vi "Get LogFile Path from SysDef.vi"(8 "error in (no error)":errorcluster, 11 "System Definition File":path) -> (0 "error out":errorcluster, 3 "Log File Path":path)   [LabVIEW 2026, in "Telemetry Test Utilities.lvlib"]
uses:
  Telemetry Test Utilities.lvlib
  Source/Shared/Constants.vi
  <vilib>/NI VeriStand/Custom Device Tools/Custom Device Utility Library/NI VeriStand - Search for Item by GUID.vi
  <vilib>/NI VeriStand/Custom Device API/Get Item Property (String Array).vi
  Source/Shared/Telemetry Shared.lvlib
  <vilib>/NI VeriStand/Custom Device Tools/Custom Device Utility Library/Custom Device Utility Library.lvlib
  <vilib>/NI VeriStand/Custom Device API/Custom Device API.lvlib
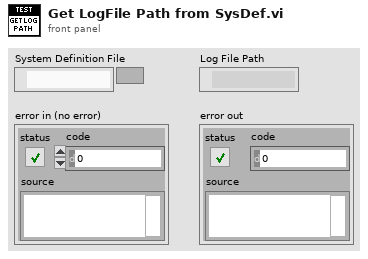
[diagram p1: front panel]
types:
  T1 = typedef "Custom Device API.lvlib/Custom Device Item Ref.ctl" = u64
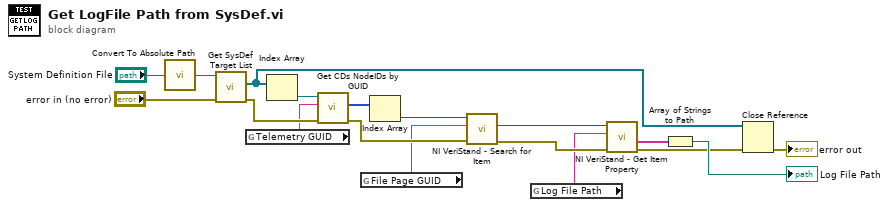
[diagram p0: block diagram]
diagram:
  n1 = call "Convert To Absolute Path.vi"("System Definition File Path"="System Definition File") -> ("Absolute path"=w4:path)
  n2 = call "Get SysDef Target List.vi"("error in (no error)"="error in (no error)", "System Definition Path"=w4) -> ("error out"=w14:errorcluster, "Target List"=w9:refnum<k24>[])  [unwired: 8 in]
  n3 = global read "Constants.vi" "Telemetry GUID"() -> (w7:string)
  n4 = Index Array(array=w9) -> (element=w6:refnum<k24>)  [unwired: 1 in]
  n5 = call "Get CDs NodeIDs by GUID.vi"("error in (no error)"=w14, "Custom Device GUID"=w7, "Target ref in"=w6) -> ("error out"=w15:errorcluster, "NodeIDs"=w8:u64[])  [unwired: 6 in, 1 out]
  n6 = global read "Constants.vi" "File Page GUID"() -> (w11:string)
  n7 = Index Array(array=w8) -> (element=w10:u64)  [unwired: 1 in]
  n8 = call-poly <vilib>:"NI VeriStand - Search for Item.vi"("error in"=w15, "Item GUID"=w11, "Section Ref in"=w10) -> ("error out"=w16:errorcluster, "Item Ref"=w12:T1)  [unwired: 5 in, 2 out]
  n9 = global read "Constants.vi" "Log File Path"() -> (w13:string)
  n10 = call-poly <vilib>:"NI VeriStand - Get Item Property.vi"("error in (no error)"=w16, "Property Name"=w13, "Item Ref in"=w12) -> ("error out"=w2:errorcluster, "Value"=w17:string[])  [unwired: 5 in, 2 out]
  n11 = Array of Strings to Path(0:w17) -> (2:→"Log File Path":path)  [unwired: 1 in]
  n12 = Close Reference(reference=w9, error in (no error)=w2) -> (error out=→"error out":errorcluster)
